vi "波形编辑.vi"(11 "connection reference":T1) -> (3 "波形图":waveform(dbl)(graph))   [LabVIEW 2020, in "功能选择.xctl"]
uses:
  <vilib>/addons/database/Connection.llb/Conn ObjectReference.ctl
  <vilib>/Utility/file.llb/Write Delimited Spreadsheet (string).vi
  <vilib>/Utility/file.llb/Read Delimited Spreadsheet (string).vi
  <vilib>/addons/database/_DB Variant To Data/Database Variant To Data.xnode
  <vilib>/addons/database/NI_Database_API.lvlib
panel:
  in  "搜索":string
  out "列表框":i32(listbox)
  in  "限流":dbl
  in  "采样点":dbl=1e-05
  in  "波形描述":string[][](table)=[["--------", "--end--", "--------", "--------"]]
  # "类型：\nL=线性  log=对数\nP=脉冲  S=阶跃"
  # "类型为对数时备注为渐近线线\n         脉冲时为占空比0-100\n         阶跃信号为突变位置0-100"
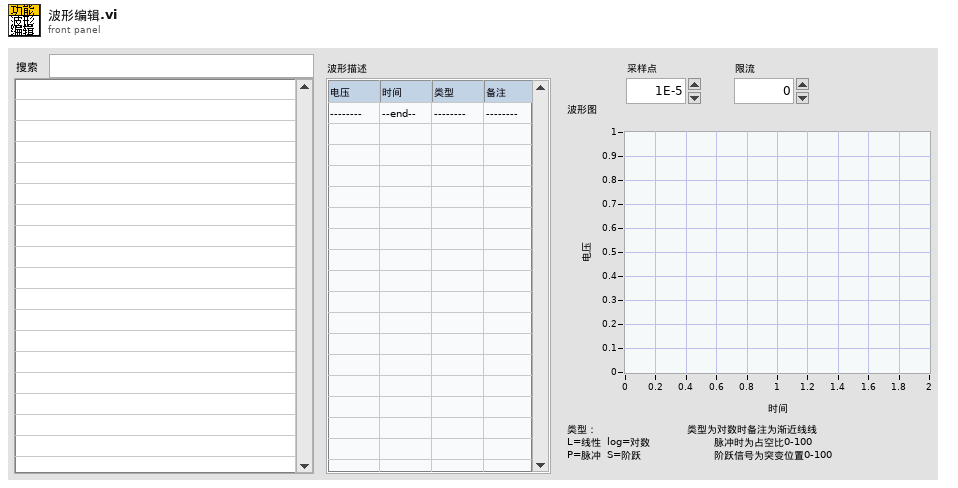
[diagram p1: front panel]
types:
  T1 = typedef "NI_Database_API.lvlib/Conn ObjectReference.ctl" = refnum<k1>
  T2 = cluster{"名称":string, "采样点":dbl, "限流":dbl, "data string":string}
  T3 = typedef "LVPoint32TypeDef.ctl" = cluster{"Horizontal":i32, "Vertical":i32}
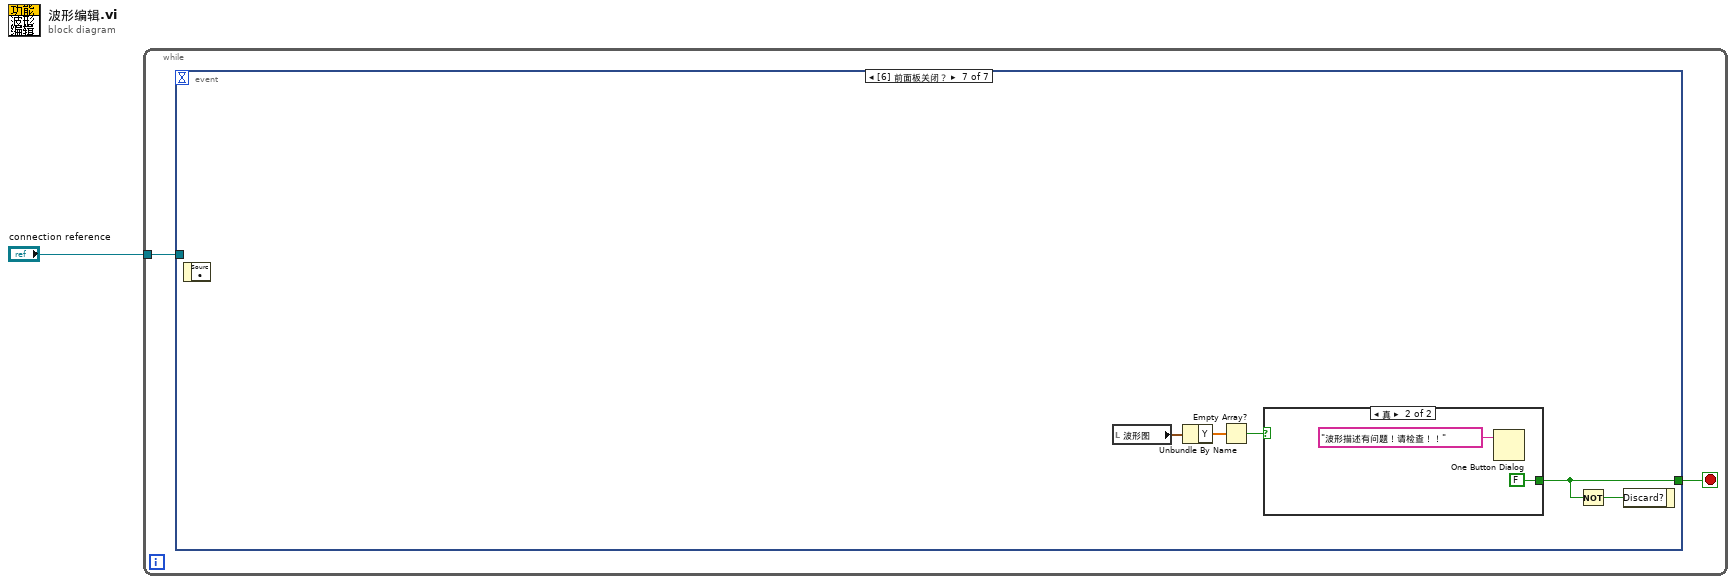
[diagram p0: block diagram]
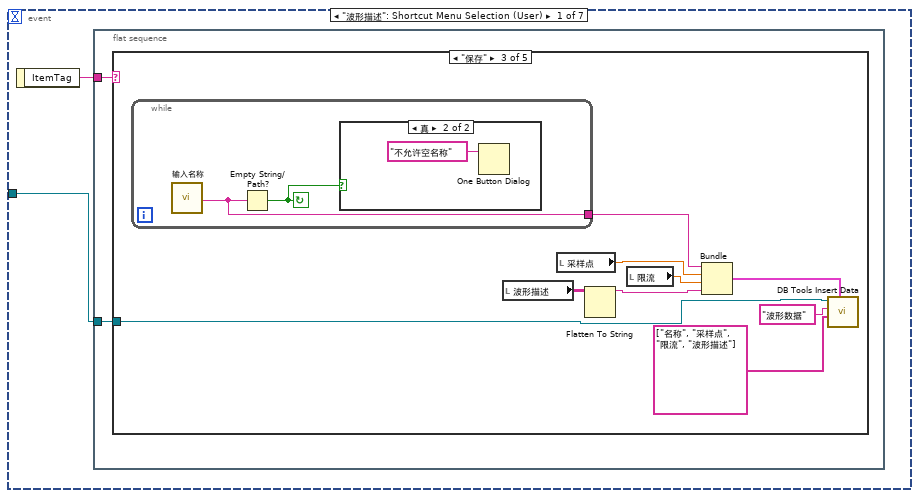
[diagram p2: hidden frame]
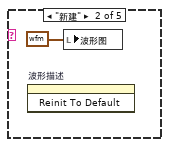
[diagram p4: hidden frame]
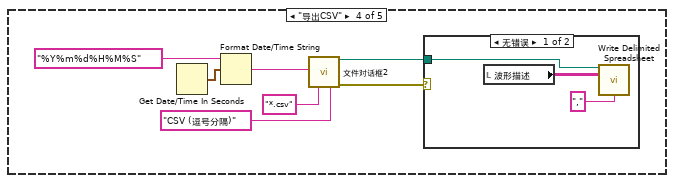
[diagram p6: hidden frame]
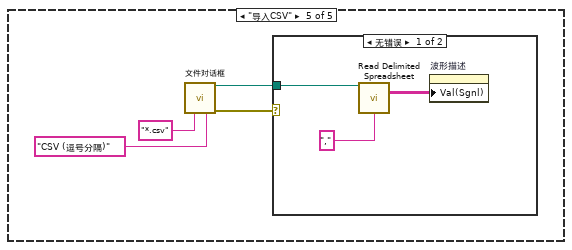
[diagram p8: hidden frame]
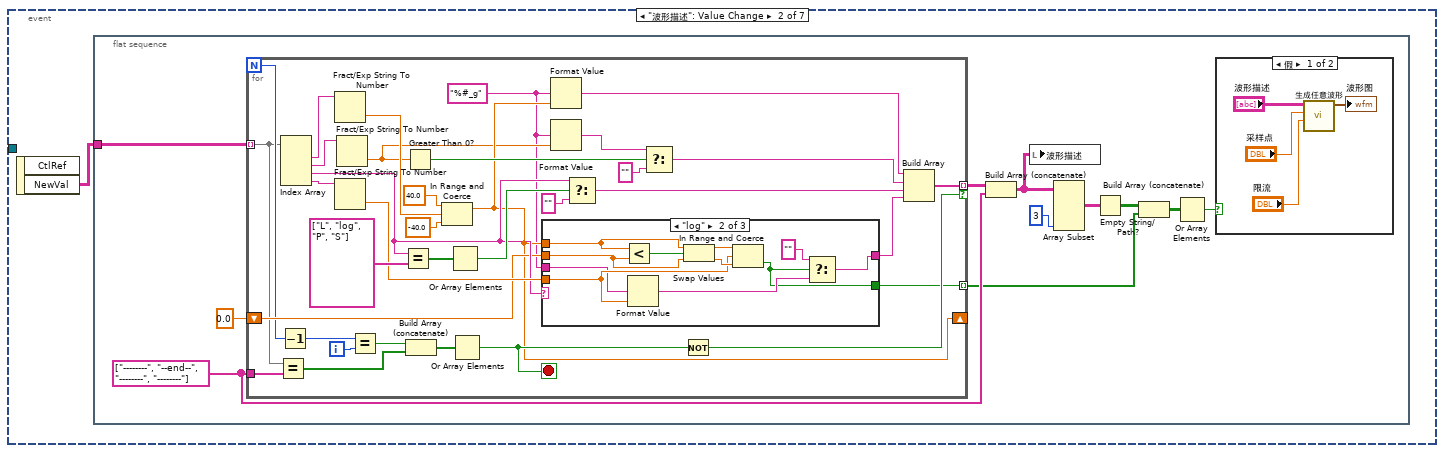
[diagram p10: hidden frame]
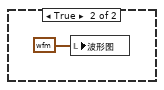
[diagram p11: hidden frame]
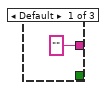
[diagram p12: hidden frame]
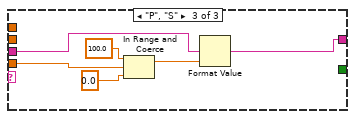
[diagram p13: hidden frame]
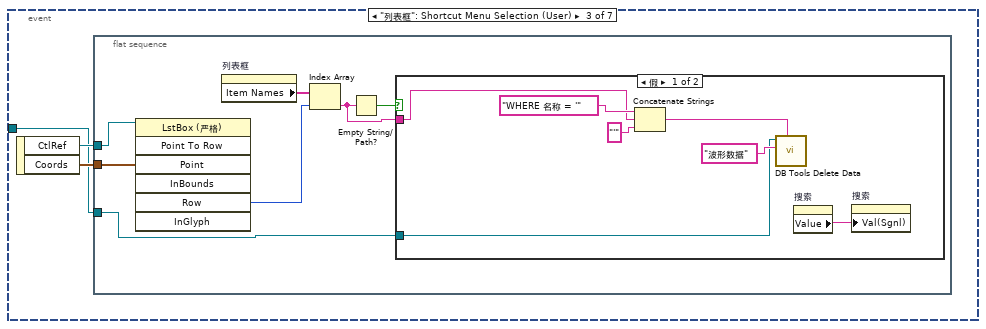
[diagram p14: hidden frame]
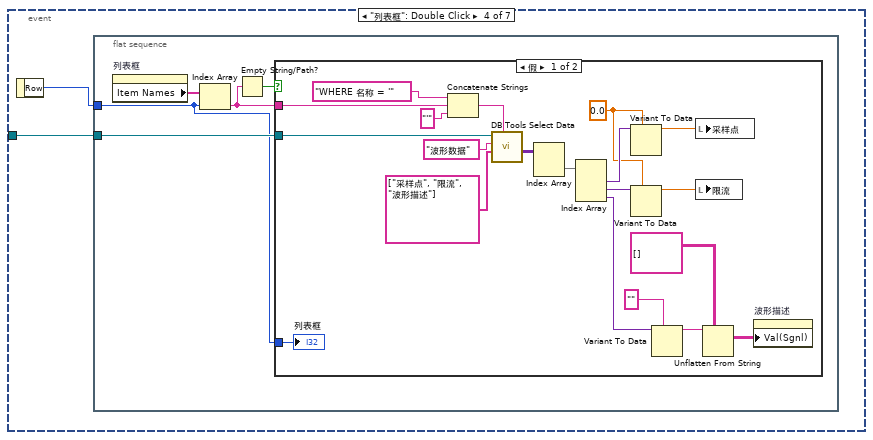
[diagram p16: hidden frame]
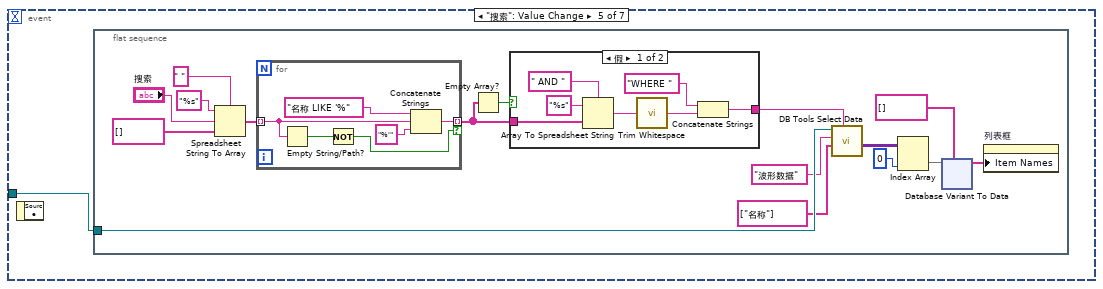
[diagram p18: hidden frame]
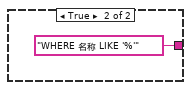
[diagram p19: hidden frame]
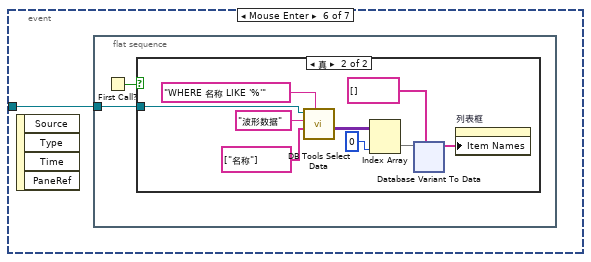
[diagram p20: hidden frame]
diagram:
  n1 = while {
    tunnel: "connection reference" -> [w2]
    stop <- w3 stop-if-true
    n2 = event shown="[6] 前面板关闭？" {
      selector: _ -> [_ _ _ _ _ _ _]
      dyn-events: _ -> [_ _ _ _ _ _ _]
      timeout: _ -> [_ _ _ _ _ _ _]
      tunnel: [_ _ _ _ _ _ w275] -> w3
      tunnel: w2 -> [w4 _ w108 w126 w152 w221 _]
      event "波形描述": Shortcut Menu Selection (User) {
        n3 = event-data() -> ("ItemTag"=w5:string)  [unwired: 1 in]
        n4 = flat-sequence {
          tunnel: w5 -> [w7]
          tunnel: w4 -> [w6]
          frame #0 {
            n5 = case shown="\"保存\"" w7 {
              tunnel: w6 -> [_ _ w14 _ _]
              frame Default {
              }
              frame "新建" {
                n6 = invoke on="波形描述" class="Tbl (严格)" method="Reinit To Default"() -> ()  [unwired: 3 in, 3 out]
                n7 = local write "波形图"(waveform(dbl) {"t0"=timestamp(0 s since 1904-01-01), "dt"=1.0, "Y"=[]} ("波形图")) -> ()
              }
              frame "保存" {
                n8 = while {
                  tunnel: [w19] -> w13
                  stop <- w18 continue-if-true
                  n9 = call "输入名称"() -> ("名称"=w19:string)  [unwired: 17 in, 2 out]
                  n10 = Empty String/Path?(string/path=w19) -> (empty?=w18:bool)
                  n11 = case shown="真" w18 {
                    frame False {
                    }
                    frame True {
                      n12 = One Button Dialog(message="不允许空名称" ("消息")) -> ()  [unwired: 1 in, 1 out]
                    }
                  }
                }
                n13 = local read "波形描述"() -> (w12:string[][])
                n14 = local read "采样点"() -> (w10:dbl)
                n15 = Flatten To String(anything=w12) -> (data string=w11:string)  [unwired: 3 in, 2 out]
                n16 = local read "限流"() -> (w9:dbl)
                n17 = Bundle("名称"=w13, "采样点"=w10, "限流"=w9, "data string"=w11) -> (w17:T2)  [unwired: 1 in]
                n18 = call <vilib>:"DB Tools Insert Data.vi"("data"=w17, "columns"=string[] ["名称", "采样点", "限流", "波形描述"], "table"="波形数据", "connection reference"=w14) -> ()  [unwired: 6 in, 2 out]
              }
              frame "导出CSV" {
                n19 = Get Date/Time In Seconds() -> (seconds since 1Jan1904=w24:timestamp)
                n20 = Format Date/Time String(time format string (%c)="%Y%m%d%H%M%S" ("时间格式字符串(%c)"), seconds (now)=w24) -> (date/time string=w23:string)  [unwired: 1 in]
                n21 = call "文件对话框2"("default name"=w23, "pattern (all files)"="*.csv" ("pattern label"), "pattern label"="CSV (逗号分隔)" ("pattern (all files)")) -> ("selected path"=w27:path, "error out"=w21:errorcluster)  [unwired: 9 in, 2 out]
                n22 = case shown="无错误" w21 {
                  tunnel: w27 -> [w30 _]
                  frame No Error {
                    n23 = local read "波形描述"() -> (w29:string[][])
                    n24 = call-poly <vilib>:"Write Delimited Spreadsheet.vi"("file path (dialog if empty)"=w30, "2D data"=w29, "delimiter (\\t)"="," ("delimiter (\\t)")) -> ()  [unwired: 11 in, 2 out]
                  }
                  frame Error {
                  }
                }
              }
              frame "导入CSV" {
                n25 = call "文件对话框"("pattern (all files)"="*.csv" ("pattern label"), "pattern label"="CSV (逗号分隔)" ("pattern (all files)")) -> ("selected path"=w34:path, "error out"=w33:errorcluster)  [unwired: 10 in, 2 out]
                n26 = case shown="无错误" w33 {
                  tunnel: w34 -> [w37 _]
                  frame No Error {
                    n27 = call-poly <vilib>:"Read Delimited Spreadsheet.vi"("file path (dialog if empty)"=w37, "delimiter (\\t)"="," ("delimiter (\\t)")) -> ("all rows"=w35:string[][])  [unwired: 8 in, 5 out]
                    n28 = property on="波形描述" class="Tbl (严格)"("Val(Sgnl)"=w35) -> ()  [unwired: 2 in, 2 out]
                  }
                  frame Error {
                  }
                }
              }
            }
          }
        }
      }
      event "波形描述": Value Change {
        n29 = event-data() -> ("NewVal"=w38:string[][])  [unwired: 1 in, 1 out]
        n30 = flat-sequence {
          tunnel: w38 -> [w49]
          frame #0 {
            w46 = string[] ["--------", "--end--", "--------", "--------"] ("波形描述")
            n31 = for {
              N -> [w65]
              tunnel: w49 -> [w58] mode=indexing
              shift-right: [w60] -> _
              shift-left: 0.0 -> [w70]
              tunnel: [w69] -> w47 mode=indexing if=w66
              tunnel: w46 -> [w57]
              tunnel: [w55] -> w39 mode=indexing
              i -> [w64]
              stop <- w67 stop-if-true
              w56 = "%#_g" ("格式字符串")
              n32 = Equal?(x=w58, y=w57) -> (x = y?=w68:bool[])
              n33 = Decrement(x=w65) -> (x-1=w63:i32)
              n34 = Index Array(array=w58) -> (element #1=w89:string, element #2=w88:string, element #3=w73:string, element #4=w87:string)  [unwired: 4 in]
              n35 = Fract/Exp String To Number(string=w89) -> (number=w71:dbl)  [unwired: 3 in, 1 out]
              n36 = Fract/Exp String To Number(string=w87) -> (number=w74:dbl)  [unwired: 3 in, 1 out]
              n37 = Fract/Exp String To Number(string=w88) -> (number=w59:dbl)  [unwired: 3 in, 1 out]
              n38 = Equal?(x=w63, y=w64) -> (x = y?=w61:bool)
              n39 = Equal?(x=w73, y=string[] ["L", "log", "P", "S"] ("NewVal")) -> (x = y?=w83:bool[])
              n40 = Greater Than 0?(x=w59) -> (x > 0?=w78:bool)
              n41 = Build Array (concatenate)(w61, w68) -> (w62:bool[])
              n42 = In Range and Coerce(upper limit=40.0 ("上限"), x=w71, lower limit=-40.0 ("下限")) -> (coerced(x)=w60:dbl)  [unwired: 1 out]
              n43 = Or Array Elements(Boolean array=w83) -> (logical OR=w82:bool)
              n44 = Or Array Elements(Boolean array=w62) -> (logical OR=w67:bool)
              n45 = case shown="\"log\"" w73 {
                tunnel: w74 -> [_ w93 w105]
                tunnel: ["" w94 w104] -> w72
                tunnel: w60 -> [_ w101 _]
                tunnel: w70 -> [_ w100 _]
                tunnel: w56 -> [_ w92 w102]
                tunnel: [_ w91 _] -> w55
                frame Default {
                }
                frame "log" {
                  n46 = Less?(x=w101, y=w100) -> (x < y?=w99:bool)
                  n47 = Format Value(format string=w92, value (0)=w93) -> (output string=w95:string)  [unwired: 1 in]
                  n48 = Swap Values(12:w101, 13:w99, 14:w100) -> (1:w97:dbl, 3:w98:dbl)
                  n49 = In Range and Coerce(upper limit=w97, x=w93, lower limit=w98) -> (In Range?=w91:bool)  [unwired: 1 out]
                  n50 = Select(t="", s=w91, f=w95) -> (s? t:f=w94:string)
                }
                frame "P", "S" {
                  n51 = In Range and Coerce(upper limit=100.0 ("上限"), x=w105, lower limit=0.0 ("下限")) -> (coerced(x)=w103:dbl)  [unwired: 1 out]
                  n52 = Format Value(format string=w102, value (0)=w103) -> (output string=w104:string)  [unwired: 1 in]
                }
              }
              n53 = Format Value(format string=w56, value (0)=w60) -> (output string=w84:string)  [unwired: 1 in]
              n54 = Format Value(format string=w56, value (0)=w59) -> (output string=w77:string)  [unwired: 1 in]
              n55 = Select(t=w73, s=w82, f="") -> (s? t:f=w79:string)
              n56 = Select(t=w77, s=w78, f="") -> (s? t:f=w75:string)
              n57 = Not(x=w67) -> (.not. x?=w66:bool)
              n58 = Build Array(w84, w75, w79, w72) -> (w69:string[])
            }
            n59 = Build Array (concatenate)(w47, w46) -> (w45:string[][])
            n60 = local write "波形描述"(w45) -> ()
            n61 = Array Subset(array=w45, length (col)=3 ("长度")) -> (w43:string[][])  [unwired: 3 in]
            n62 = Empty String/Path?(string/path=w43) -> (empty?=w42:bool[][])
            n63 = Build Array (concatenate)(w42, w39) -> (w40:bool[][])
            n64 = Or Array Elements(Boolean array=w40) -> (logical OR=w41:bool)
            n65 = case shown="假" w41 {
              frame False {
                n66 = call "生成任意波形.vi"("限流"="限流", "采样点"="采样点", "波形描述"="波形描述") -> ("波形图"=→"波形图":waveform(dbl))  [unwired: 8 in]
              }
              frame True {
                n67 = local write "波形图"(waveform(dbl) {"t0"=timestamp(0 s since 1904-01-01), "dt"=1.0, "Y"=[]} ("Waveform")) -> ()
              }
            }
          }
        }
      }
      event "列表框": Shortcut Menu Selection (User) {
        n68 = event-data() -> ("CtlRef"=w110:refnum<vi>, "Coords"=w109:T3)  [unwired: 1 in]
        n69 = flat-sequence {
          tunnel: w110 -> [w117]
          tunnel: w109 -> [w116]
          tunnel: w108 -> [w111]
          frame #0 {
            n70 = invoke class="LstBox (严格)" method="Point To Row"(reference=w117, "Point"=w116) -> ("Row"=w114:i32)  [unwired: 5 in, 6 out]
            n71 = property on="列表框" class="LstBox (严格)"() -> ("Item Names"=w115:string[])  [unwired: 2 in, 2 out]
            n72 = Index Array(array=w115, index=w114) -> (element=w113:string)
            n73 = Empty String/Path?(string/path=w113) -> (empty?=w112:bool)
            n74 = case shown="假" w112 {
              tunnel: w113 -> [w122 _]
              tunnel: w111 -> [w119 _]
              frame False {
                n75 = Concatenate Strings("WHERE 名称 = '" ("condition"), w122, "'" ("字符串")) -> (w120:string)
                n76 = call <vilib>:"DB Tools Delete Data.vi"("condition"=w120, "table"="波形数据", "connection reference"=w119) -> ()  [unwired: 7 in, 2 out]
                n77 = property on="搜索" class="Str"() -> ("Value"=w118:string)  [unwired: 2 in, 2 out]
                n78 = property on="搜索" class="Str"("Val(Sgnl)"=w118) -> ()  [unwired: 2 in, 2 out]
              }
              frame True {
              }
            }
          }
        }
      }
      event "列表框": Double Click {
        n79 = event-data() -> ("Row"=w125:i32)  [unwired: 1 in]
        n80 = flat-sequence {
          tunnel: w126 -> [w131]
          tunnel: w125 -> [w130]
          frame #0 {
            n81 = property on="列表框" class="LstBox (严格)"() -> ("Item Names"=w129:string[])  [unwired: 2 in, 2 out]
            n82 = Index Array(array=w129, index=w130) -> (element=w128:string)
            n83 = Empty String/Path?(string/path=w128) -> (empty?=w127:bool)
            n84 = case shown="假" w127 {
              tunnel: w131 -> [w151 _]
              tunnel: w130 -> [w135 _]
              tunnel: w128 -> [w134 _]
              frame False {
                w141 = 0.0
                n85 = Concatenate Strings("WHERE 名称 = '" ("condition"), w134, "'" ("字符串")) -> (w147:string)
                n86 = call <vilib>:"DB Tools Select Data.vi"("condition"=w147, "columns"=string[] ["采样点", "限流", "波形描述"], "table"="波形数据", "connection reference"=w151) -> ("data"=w146:variant[][])  [unwired: 2 in, 2 out]
                n87 = Index Array(array=w146) -> (element=w145:variant[])  [unwired: 2 in]
                n88 = Index Array(array=w145) -> (element #1=w144:variant, element #2=w142:variant, element #3=w138:variant)  [unwired: 3 in]
                n89 = Variant To Data(type=w141, Variant=w144) -> (data=w143:dbl)  [unwired: 1 in, 1 out]
                n90 = Variant To Data(type=w141, Variant=w142) -> (data=w140:dbl)  [unwired: 1 in, 1 out]
                n91 = Variant To Data(type="", Variant=w138) -> (data=w139:string)  [unwired: 1 in, 1 out]
                n92 = local write "采样点"(w143) -> ()
                n93 = local write "限流"(w140) -> ()
                n94 = Unflatten From String(type=string[][] [], binary string=w139) -> (value=w132:string[][])  [unwired: 3 in, 2 out]
                n95 = property on="波形描述" class="Tbl (严格)"("Val(Sgnl)"=w132) -> ()  [unwired: 2 in, 2 out]
                "列表框" <- w135
              }
              frame True {
              }
            }
          }
        }
      }
      event "搜索": Value Change {
        n96 = event-data() -> ()  [unwired: 1 in, 1 out]
        n97 = flat-sequence {
          tunnel: w152 -> [w167]
          frame #0 {
            n98 = Spreadsheet String To Array(delimiter (Tab)=" " ("分隔符(Tab)"), format string="%s" ("格式字符串"), spreadsheet string="搜索", array type (2D Dbl)=string[] []) -> (array=w155:string[])
            n99 = for {
              tunnel: w155 -> [w179] mode=indexing
              tunnel: [w180] -> w154 mode=indexing if=w177
              n100 = Empty String/Path?(string/path=w179) -> (empty?=w178:bool)
              n101 = Not(x=w178) -> (.not. x?=w177:bool)
              n102 = Concatenate Strings("名称 LIKE '%" ("字符串"), w179, "%'" ("condition")) -> (w180:string)
            }
            n103 = Empty Array?(array=w154) -> (empty?=w153:bool)
            n104 = case shown="假" w153 {
              tunnel: [w171 "WHERE 名称 LIKE '%'"] -> w159
              tunnel: w154 -> [w169 _]
              frame False {
                n105 = Array To Spreadsheet String(delimiter (Tab)=" AND " ("分隔符(Tab)"), array=w169, 3:"%s" ("格式字符串")) -> (spreadsheet string=w173:string)
                n106 = call <vilib>:"Trim Whitespace.vi"("string"=w173) -> ("trimmed string"=w172:string)  [unwired: 1 in]
                n107 = Concatenate Strings("WHERE ", w172) -> (w171:string)
              }
              frame True {
              }
            }
            n108 = call <vilib>:"DB Tools Select Data.vi"("condition"=w159, "columns"=string[] ["名称"], "table"="波形数据", "connection reference"=w167) -> ("data"=w164:variant[][])  [unwired: 2 in, 2 out]
            n109 = Index Array(array=w164, index (col)=0 ("禁用的索引 (列)")) -> (element=w163:variant[])  [unwired: 1 in]
            n110 = xnode "Database Variant To Data"("database variant"=w163, "type"=string[] [] ("数据")) -> ("data"=w161:string[])  [unwired: 1 in, 1 out]
            n111 = property on="列表框" class="LstBox (严格)"("Item Names"=w161) -> ()  [unwired: 2 in, 2 out]
          }
        }
      }
      event Mouse Enter {
        n112 = event-data() -> ()  [unwired: 1 in, 4 out]
        n113 = flat-sequence {
          tunnel: w221 -> [w222]
          frame #0 {
            n114 = First Call?() -> (First Call?: T/F=w223:bool)
            n115 = case shown="真" w223 {
              tunnel: w222 -> [_ w224]
              frame False {
              }
              frame True {
                n116 = call <vilib>:"DB Tools Select Data.vi"("condition"="WHERE 名称 LIKE '%'", "columns"=string[] ["名称"], "table"="波形数据", "connection reference"=w224) -> ("data"=w232:variant[][])  [unwired: 2 in, 2 out]
                n117 = Index Array(array=w232, index (col)=0 ("禁用的索引 (列)")) -> (element=w231:variant[])  [unwired: 1 in]
                n118 = xnode "Database Variant To Data"("database variant"=w231, "type"=string[] [] ("数据")) -> ("data"=w230:string[])  [unwired: 1 in, 1 out]
                n119 = property on="列表框" class="LstBox (严格)"("Item Names"=w230) -> ()  [unwired: 2 in, 2 out]
              }
            }
          }
        }
      }
      event Panel Close? {
        n120 = event-data() -> ()  [unwired: 1 in, 1 out]
        n121 = local read "波形图"() -> (w273:waveform(dbl))
        n122 = Unbundle By Name(w273) -> ("Y"=w272:dbl[])
        n123 = Empty Array?(array=w272) -> (empty?=w271:bool)
        n124 = case shown="真" w271 {
          tunnel: [w276 FALSE ("T button?")] -> w275
          frame False {
            n125 = Two Button Dialog(message="确定？" ("消息")) -> (T button?=w276:bool)  [unwired: 2 in]
          }
          frame True {
            n126 = One Button Dialog(message="波形描述有问题！请检查！！" ("消息")) -> ()  [unwired: 1 in, 1 out]
          }
        }
        n127 = Not(x=w275) -> (.not. x?=w274:bool)
        n128 = event-data("Discard?"=w274) -> ()  [unwired: 1 in, 1 out]
      }
    }
  }
